vi "Pointer Class Name.vi"() -> (3 "pointer class name":string="Pointer")   [LabVIEW 2027, in "Memory Manager.lvlib"]
doc: "A set of block diagram constants used throughout this library."
uses:
  Memory Manager.lvlib
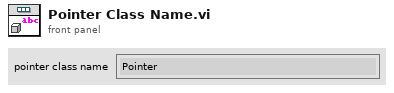
[diagram p1: front panel]
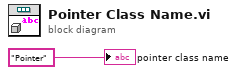
[diagram p0: block diagram]
diagram:
  "pointer class name" <- "Pointer"
